vi "Write String to Temp File.vi"(8 "error in":errorcluster, 10 "file extension in":string, 11 "string in":string) -> (0 "error out":errorcluster, 3 "file path out":path)   [LabVIEW 2019]
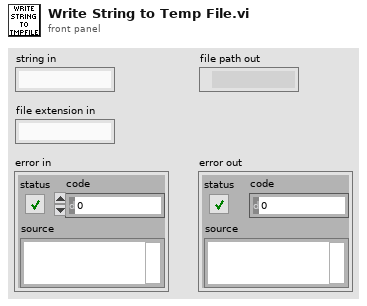
[diagram p1: front panel]
types:
  T1 = enum16{"open", "replace", "create", "open or create", "replace or create", "replace or create with confirmation"}
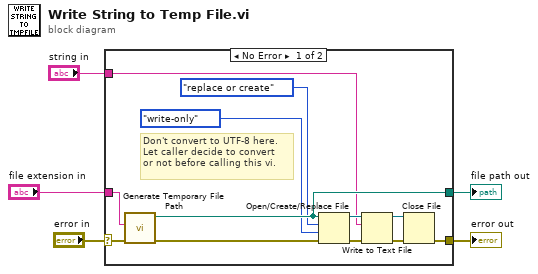
[diagram p0: block diagram]
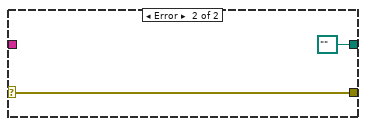
[diagram p2: hidden frame]
diagram:
  n1 = case shown="No Error" "error in" {
    selector: "error in" -> [w7 w19]
    tunnel: "string in" -> [w6 _]
    tunnel: [w17 w19] -> w4
    tunnel: [w16 path "" ("Unique Temporary File Path")] -> w3
    tunnel: "file extension in" -> [w10 _]
    frame No Error {
      # "Don't convert to UTF-8 here.\nLet caller decide to convert\nor not before calling this vi."
      n2 = call <vilib>:"Generate Temporary File Path.vi"("error in (no error)"=w7, "Temporary File Extension (tmp)"=w10) -> ("error out"=w8:errorcluster, "Unique Temporary File Path"=w16:path)  [unwired: 8 in]
      n3 = Open/Create/Replace File(file path (use dialog)=w16, error in=w8, operation (0:open)=T1."replace or create", access (0:read/write)=enum16{"read/write", "read-only", "write-only"}."write-only") -> (refnum out=w13:refnum<file>, error out=w9:errorcluster)  [unwired: 2 in, 1 out]
      n4 = Write to Text File(file (use dialog)=w13, text=w6, error in=w9) -> (refnum out=w12:refnum<file>, error out=w11:errorcluster)  [unwired: 1 in, 1 out]
      n5 = Close File(refnum=w12, error in=w11) -> (error out=w17:errorcluster)  [unwired: 1 out]
    }
    frame Error {
    }
  }
  "error out" <- w4
  "file path out" <- w3
